vi "RDS Serial Handler Close.vi"(8 "error in (no error)":errorcluster, 11 "RDS Serial Instrument in":refnum<class "RDS Serial Instrument.lvclass">) -> (0 "error out":errorcluster, 3 "RDS Serial Instrument out":refnum<class "RDS Serial Instrument.lvclass">)   [LabVIEW 2015, in "RDS Serial Handler.lvlib" / "RDS Serial Instrument.lvclass"]
uses:
  RDS Serial Instrument.lvclass
  RDS Serial Instrument.lvclass/RDS Serial Instrument.ctl
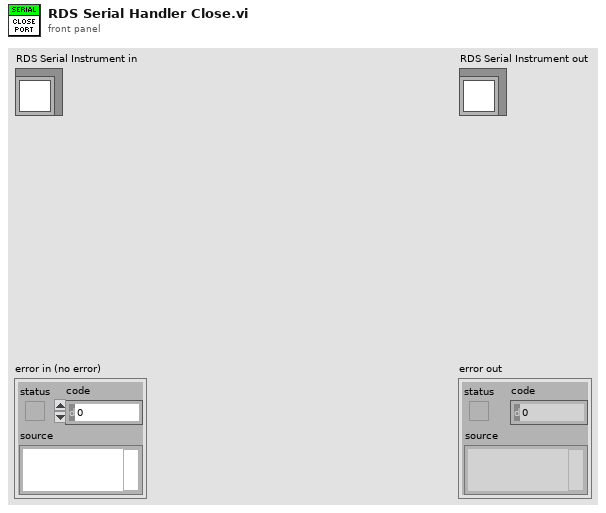
[diagram p1: front panel]
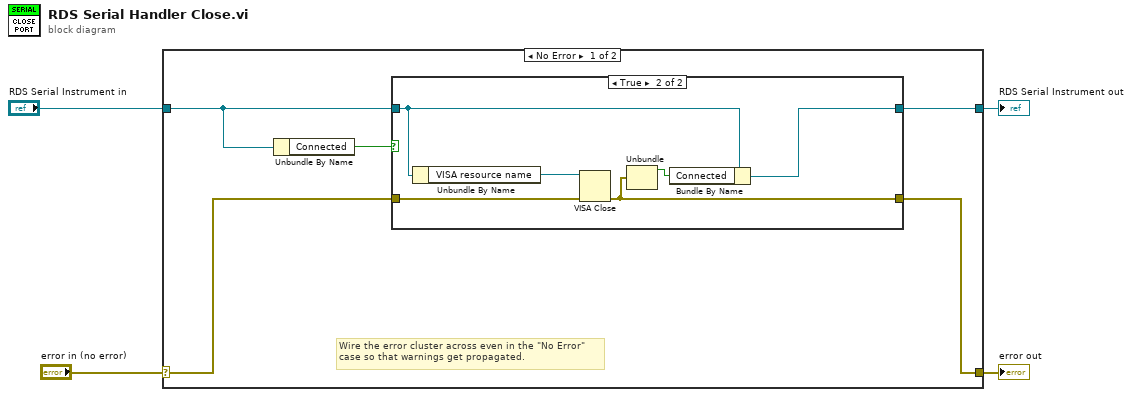
[diagram p0: block diagram]
diagram:
  n1 = case shown="No Error" "error in (no error)" {
    selector: "error in (no error)" -> [w9 w19]
    tunnel: [w7 w19] -> w3
    tunnel: [w8 w18] -> w1
    tunnel: "RDS Serial Instrument in" -> [w6 w18]
    frame No Error {
      # "Wire the error cluster across even in the \"No Error\"\ncase so that warnings get propagated."
      n2 = Unbundle By Name(w6) -> ("Connected"=w5:bool)
      n3 = case shown="True" w5 {
        tunnel: w9 -> [w10 w16]
        tunnel: w6 -> [w11 w15]
        tunnel: [w11 w14] -> w8
        tunnel: [w10 w13] -> w7
        frame False {
        }
        frame True {
          n4 = Unbundle By Name(w15) -> ("VISA resource name"=w17:refnum<visa-resource-name>)
          n5 = VISA Close(VISA resource name=w17, error in (no error)=w16) -> (error out=w13:errorcluster)
          n6 = Unbundle(w13) -> ("status"=w12:bool)  [unwired: 2 out]
          n7 = Bundle By Name(cluster=w15, "Connected"=w12) -> (w14:refnum<class "RDS Serial Instrument.lvclass">)
        }
      }
    }
    frame Error {
    }
  }
  "error out" <- w3
  "RDS Serial Instrument out" <- w1
